vi "Execute.vi"(5 "SleepTerminalArray":refnum<vi>, 6 "ExeRef":refnum<vi>, 7 "ActiveTerminalArray":refnum<vi>, 8 "error in (no error)":errorcluster, 9 "Json_In":string, 10 "VariableRef":T2, 11 "Info":T1) -> (0 "Error Out":errorcluster, 1 "NumResultArray":dbl[](array[numeric]), 2 "StrResultArray":string[](array[string]), 3 "StrResult":string, 4 "NumResult":dbl)   [LabVIEW 2018, in "Time.lvlib"]
uses:
  Time.lvlib
  <userlib>/_OpenG.lib/dictionary/dictionary.llb/Dictionary Object RefNum__ogtk.ctl
  <userlib>/_OpenG.lib/dictionary/dictionary.llb/Dictionary Object RefNum - Enum__ogtk.ctl
  <userlib>/_MGI/Timing/MGI Wait/MGI Wait (U32).vi
  <vilib>/addons/_JKI.lib/Serialization/JSON/JKI JSON Serialization.lvlib
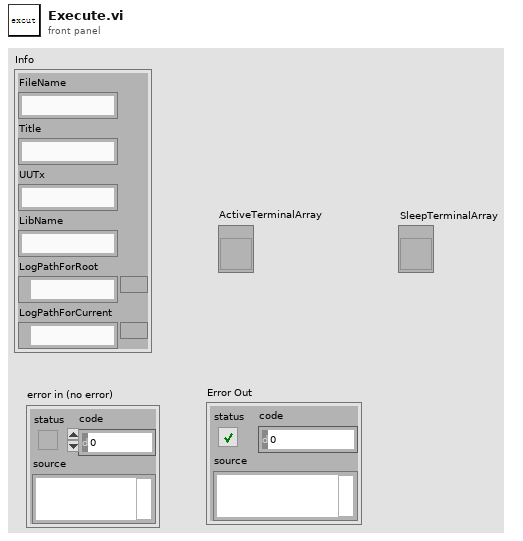
[diagram p1: front panel]
types:
  T1 = cluster{"FileName":string, "Title":string, "UUTx":string, "LibName":string, "LogPathForRoot":path, "LogPathForCurrent":path}
  T2 = typedef "Dictionary Object RefNum__ogtk.ctl" = refnum<k1>
  T3 = cluster{"Wait_ms":cluster{"json":cluster{"Method":string, "Time":i32}}, "Wait_s":cluster{"json":cluster{"Method":string, "Time":i32}}, "TickCount":cluster{"json":cluster{"Method":string}}}
  T4 = cluster{"json":cluster{"Method":string, "Time":i32}}
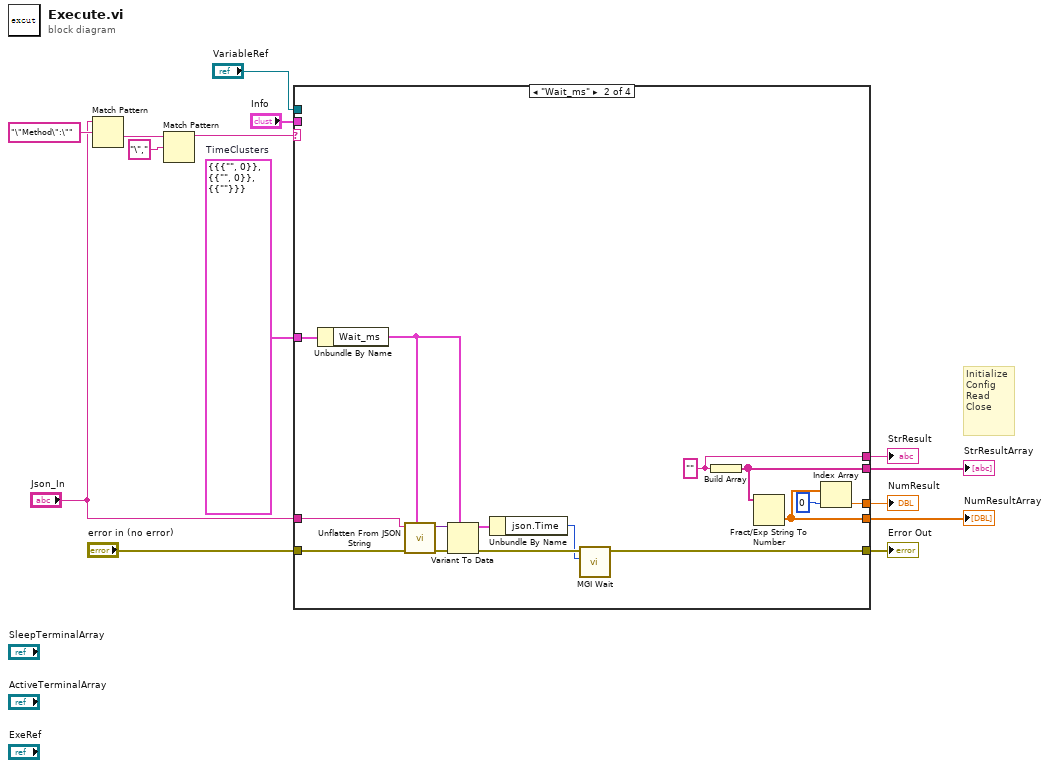
[diagram p0: block diagram]
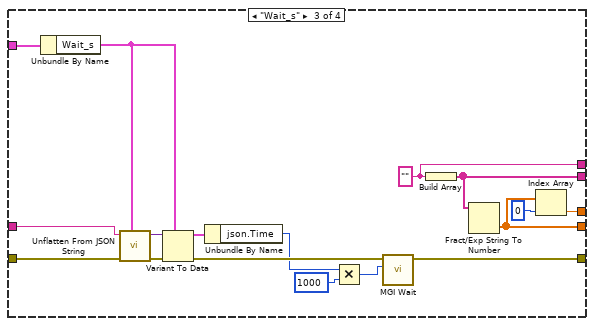
[diagram p3: hidden frame]
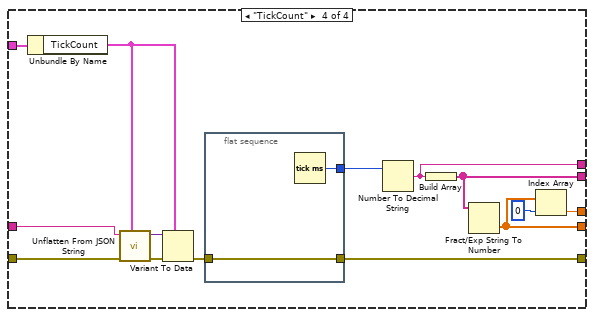
[diagram p4: hidden frame]
diagram:
  w1 = T3 {"Wait_ms"={"json"={"Method"="", "Time"=0}}, "Wait_s"={"json"={"Method"="", "Time"=0}}, "TickCount"={"json"={"Method"=""}}}  # TimeClusters
  # "Initialize\nConfig\nRead\nClose"
  n1 = Match Pattern(string="Json_In", regular expression="\"Method\":\"") -> (after substring=w4:string)  [unwired: 1 in, 3 out]
  n2 = Match Pattern(string=w4, regular expression="\",") -> (before substring=w2:string)  [unwired: 1 in, 3 out]
  n3 = case shown="\"Wait_ms\"" w2 {
    tunnel: "Json_In" -> [_ w27 w44 w59]
    tunnel: [w15 w18 w35 w51] -> w14
    tunnel: "error in (no error)" -> [w15 w26 w43 w58]
    tunnel: [_ w16 w34 w48] -> w12
    tunnel: "VariableRef" -> [_ _ _ _]
    tunnel: [_ w20 w37 w52] -> w11
    tunnel: [_ w23 w40 w55] -> w10
    tunnel: [_ w25 w42 w57] -> w9
    tunnel: "Info" -> [_ _ _ _]
    tunnel: w1 -> [_ w22 w39 w54]
    frame Default {
    }
    frame "Wait_ms" {
      w16 = ""
      n4 = Unbundle By Name(w22) -> ("Wait_ms"=w21:T4)
      n5 = call <vilib>:"Unflatten From JSON String.vi"("Type and Defaults"=w21, "error in (no error)"=w26, "JSON String"=w27) -> ("error out"=w29:errorcluster, "Variant"=w30:variant)  [unwired: 7 in]
      n6 = Variant To Data(error in=w29, type=w21, Variant=w30) -> (data=w28:T4, error out=w19:errorcluster)
      n7 = Unbundle By Name(w28) -> ("json.Time"=w17:i32)
      n8 = call-poly <userlib>:"MGI Wait.vi"("ms"=w17, "Error In"=w19) -> ("Error Out"=w18:errorcluster)  [unwired: 5 in]
      n9 = Build Array(w16) -> (w20:string[])
      n10 = Fract/Exp String To Number(string=w20) -> (number=w25:dbl[])  [unwired: 3 in, 1 out]
      n11 = Index Array(array=w25, index=0) -> (element=w23:dbl)
    }
    frame "Wait_s" {
      w34 = ""
      n12 = Unbundle By Name(w39) -> ("Wait_s"=w38:T4)
      n13 = call <vilib>:"Unflatten From JSON String.vi"("Type and Defaults"=w38, "error in (no error)"=w43, "JSON String"=w44) -> ("error out"=w46:errorcluster, "Variant"=w47:variant)  [unwired: 7 in]
      n14 = Variant To Data(error in=w46, type=w38, Variant=w47) -> (data=w45:T4, error out=w36:errorcluster)
      n15 = Unbundle By Name(w45) -> ("json.Time"=w33:i32)
      n16 = Multiply(x=w33, y=1000) -> (x*y=w31:i32)
      n17 = call-poly <userlib>:"MGI Wait.vi"("ms"=w31, "Error In"=w36) -> ("Error Out"=w35:errorcluster)  [unwired: 5 in]
      n18 = Build Array(w34) -> (w37:string[])
      n19 = Fract/Exp String To Number(string=w37) -> (number=w42:dbl[])  [unwired: 3 in, 1 out]
      n20 = Index Array(array=w42, index=0) -> (element=w40:dbl)
    }
    frame "TickCount" {
      n21 = Unbundle By Name(w54) -> ("TickCount"=w53:cluster{"json":cluster{"Method":string}})
      n22 = call <vilib>:"Unflatten From JSON String.vi"("Type and Defaults"=w53, "error in (no error)"=w58, "JSON String"=w59) -> ("error out"=w60:errorcluster, "Variant"=w61:variant)  [unwired: 7 in]
      n23 = Variant To Data(error in=w60, type=w53, Variant=w61) -> (error out=w50:errorcluster)  [unwired: 1 out]
      n24 = flat-sequence {
        tunnel: [w63] -> w51
        tunnel: w50 -> [w63]
        tunnel: [w62] -> w49
        frame #0 {
          n25 = Tick Count (ms)() -> (millisecond timer value=w62:u32)
        }
      }
      n26 = Number To Decimal String(number=w49) -> (decimal integer string=w48:string)  [unwired: 1 in]
      n27 = Build Array(w48) -> (w52:string[])
      n28 = Fract/Exp String To Number(string=w52) -> (number=w57:dbl[])  [unwired: 3 in, 1 out]
      n29 = Index Array(array=w57, index=0) -> (element=w55:dbl)
    }
  }
  "StrResult" <- w12
  "Error Out" <- w14
  "StrResultArray" <- w11
  "NumResult" <- w10
  "NumResultArray" <- w9
